vi "Plot Descr Read.vi"(4 "error in (no error)":errorcluster, 6 "Container State":T3, 7 "Display State In":T2) -> (0 "error out":errorcluster, 2 "Value":T1(array[cluster]), 3 "Display State Out":T2)   [LabVIEW 2015, in "Tau.xctl"]
uses:
  Tau.xctl
  <vilib>/_xctls/Container State.ctl
  State.ctl
  <vilib>/_xctls/XControlSupport.lvlib
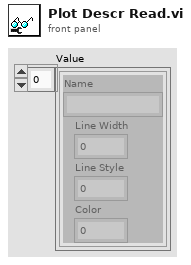
[diagram p1: front panel]
types:
  T1 = cluster{"Name":string, "Line Width":u8, "Line Style":u8, "Color":u32}[]
  T2 = typedef "Tau.xctl/State.ctl" = cluster{"Data Array":sgl[][], "Time Array":timestamp[], "History":u16, "Variable":bool[], "Plot Details":cluster{"Name":string, "Line Width":u8, "Line Style":u8, "Color":u32}[]}
  T3 = typedef "XControlSupport.lvlib/Container State.ctl" = cluster{"Indicator?":bool, "Run Mode?":bool, " Refnum":refnum<vi>}
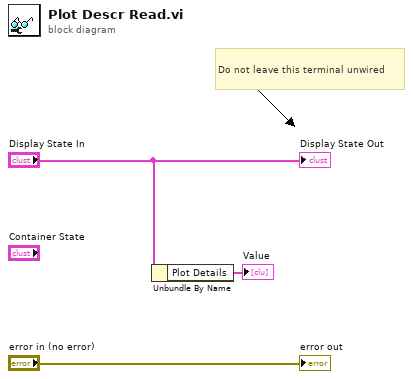
[diagram p0: block diagram]
diagram:
  # "Do not leave this terminal unwired"
  n1 = Unbundle By Name("Display State In") -> ("Plot Details"=→"Value":T1)
  "error out" <- "error in (no error)"
  "Display State Out" <- "Display State In"
